vi "Encoder_GetEncoderControlReference.vi"(2 "MotorIndex":T6, 3 "RobotEncoderRef":T5) -> (0 "Max Speed":dbl format="%#_13g", 1 "EncoderDevRef":T1={"DevStatus"={"status"=FALSE, "code"=0, "source"=""}, "EncoderIndex"=enum."Invalid", "CounterIndex"=enum."Ctr 1", "DistancePerCount"=2.0, "Decoding Type"=enum."4x"})   [LabVIEW 2013]
uses:
  <vilib>/Rock Robotics/WPI/Encoder/WPI_EncoderDevRef.ctl
  <vilib>/Rock Robotics/SystemInterfaces/Encoder/FPGA_EncoderIdx.ctl
  <vilib>/Rock Robotics/SystemInterfaces/Counter/FPGA_CounterCtrSystemIndex.ctl
  <vilib>/Rock Robotics/WPI/Encoder/WPI_EncoderType.ctl
  <vilib>/Rock Robotics/WPI/RobotDrive/WPI_RobotDriveMotorSelectorEnum.ctl
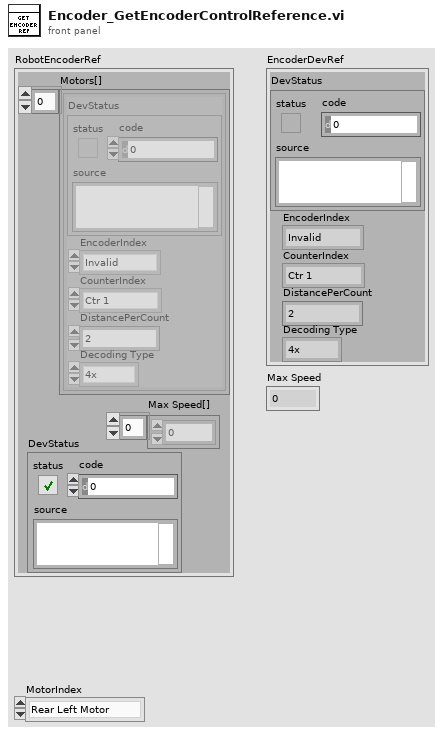
[diagram p1: front panel]
types:
  T1 = typedef "WPI_EncoderDevRef.ctl" = cluster{"DevStatus":errorcluster, "EncoderIndex":T2, "CounterIndex":T3, "DistancePerCount":dbl, "Decoding Type":T4}
  T2 = typedef "FPGA_EncoderIdx.ctl" = enum8{"Enc 0", "Enc 1", "Enc 2", "Enc 3", "Invalid"}
  T3 = typedef "FPGA_CounterCtrSystemIndex.ctl" = enum8{"Ctr 0", "Ctr 1", "Ctr 2", "Ctr 3", "Ctr 4", "Ctr 5", "Ctr 6", "Ctr 7", "Invalid"}
  T4 = typedef "WPI_EncoderType.ctl" = enum16{"1x", "2x", "4x"}
  T5 = cluster{"Motors[]":T1[], "DevStatus":errorcluster, "Max Speed[]":dbl[]}
  T6 = typedef "WPI_RobotDriveMotorSelectorEnum.ctl" = enum16{"Rear Left Motor", "Rear Right Motor", "Front Left Motor", "Front Right Motor"}
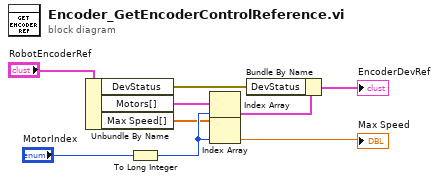
[diagram p0: block diagram]
diagram:
  n1 = Unbundle By Name("RobotEncoderRef") -> ("DevStatus"=w7:errorcluster, "Motors[]"=w9:T1[], "Max Speed[]"=w2:dbl[])
  n2 = To Long Integer(number="MotorIndex") -> (32bit integer=w3:i32)
  n3 = Index Array(array=w9, index=w3) -> (element=w8:T1)
  n4 = Index Array(array=w2, index=w3) -> (element=→"Max Speed":dbl)
  n5 = Bundle By Name(cluster=w8, "DevStatus"=w7) -> (→"EncoderDevRef":T1)
